vi "Procces coins.vi"(8 "error in (no error)":errorcluster, 10 "Coins":T1, 11 "MXN Actor in":refnum<class "MXN Actor.lvclass">) -> (0 "error out":errorcluster, 3 "MXN Actor out":refnum<class "MXN Actor.lvclass">)   [LabVIEW 2020, in "MXN Actor.lvlib" / "MXN Actor.lvclass"]
uses:
  MXN Actor.lvclass
  C:/Program Files (x86)/National Instruments/LabVIEW 2020/vi.lib/ActorFramework/Actor/Actor.lvclass
  <vilib>/ActorFramework/Actor/Actor.lvclass/Actor.ctl
  MXN Actor.lvclass/MXN Actor.ctl
  UI Actor Messages/Credit Update Msg/Credit Update Msg.lvclass/Credit Update Msg.ctl
  <vilib>/ActorFramework/Message Enqueuer/Message Enqueuer.lvclass/Message Enqueuer.ctl
  <vilib>/ActorFramework/Message Enqueuer/Enqueue.vi
  UI Actor Messages/Credit Update Msg/Credit Update Msg.lvclass
  C:/Program Files (x86)/National Instruments/LabVIEW 2020/vi.lib/ActorFramework/Message/Message.lvclass
  <vilib>/ActorFramework/Message Priority Queue/Priority Enqueue.vi
  <vilib>/ActorFramework/Actor/Actor.lvclass
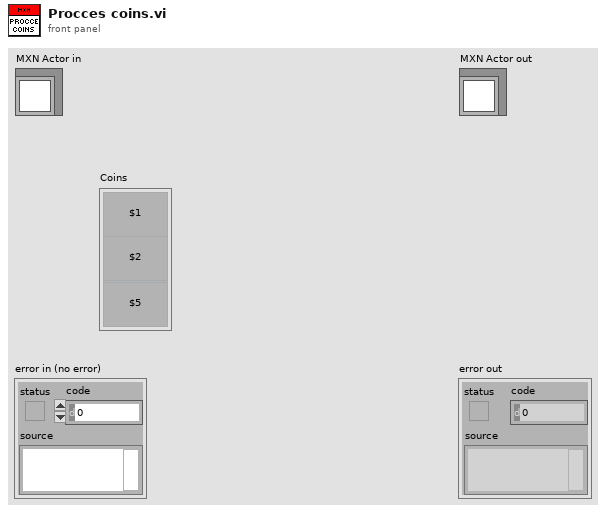
[diagram p1: front panel]
types:
  T1 = cluster{"Button":bool, "Button 2":bool, "Button 3":bool}
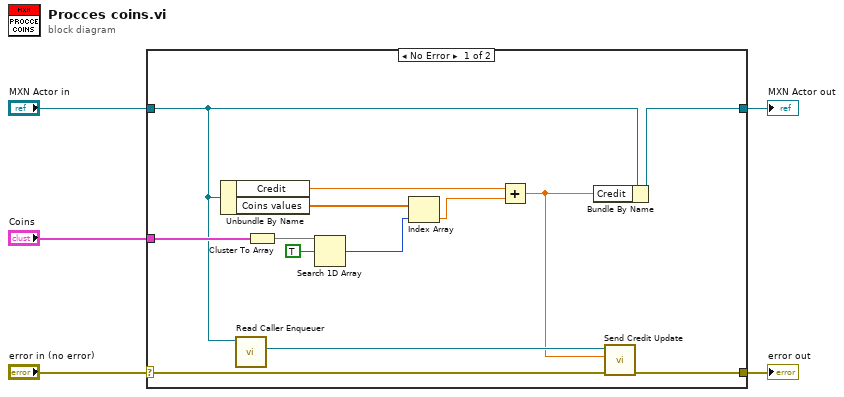
[diagram p0: block diagram]
diagram:
  n1 = case shown="No Error" "error in (no error)" {
    selector: "error in (no error)" -> [w8 w20]
    tunnel: [w7 w20] -> w4
    tunnel: [w15 w19] -> w2
    tunnel: "MXN Actor in" -> [w10 w19]
    tunnel: "Coins" -> [w14 _]
    frame No Error {
      n2 = Unbundle By Name(w10) -> ("Credit"=w16:dbl, "Coins values"=w13:dbl[])
      n3 = call <vilib>:"Read Caller Enqueuer.vi"("Actor"=w10) -> ("Caller Enqueuer"=w9:refnum<class "Message Enqueuer.lvclass">)  [unwired: 10 in]
      n4 = Cluster To Array(cluster=w14) -> (array=w18:bool[])
      n5 = Search 1D Array(1D array=w18, element=TRUE) -> (index of element=w17:i32)  [unwired: 1 in]
      n6 = Index Array(array=w13, index=w17) -> (element=w12:dbl)
      n7 = Add(x=w16, y=w12) -> (x+y=w6:dbl)
      n8 = Bundle By Name(cluster=w10, "Credit"=w6) -> (w15:refnum<class "MXN Actor.lvclass">)
      n9 = call "Send Credit Update.vi"("error in (no error)"=w8, "Credit"=w6, "Message Enqueuer"=w9) -> ("error out"=w7:errorcluster)  [unwired: 7 in, 1 out]
    }
    frame Error {
    }
  }
  "error out" <- w4
  "MXN Actor out" <- w2
